vi "Tracking_SavePoint.vi"(8 "error in":errorcluster, 10 "Image Data":T4 {"Frame Data"."Image Type" items=["Grayscale (U8)", "Grayscale (I16)", "Grayscale (SGL)", "Complex (CSG)", "RGB (U32)", "HSL (U32)", "RGB (U64)", "Grayscale (U16)"]}, 11 "Recording Data In":T1) -> (0 "error out":errorcluster)   [LabVIEW 2017, in "ImageAcquisitionLibrary.lvlib"]
uses:
  ImageAcquisitionLibrary.lvlib
  Acquisition/AcquireData.ctl
  Recording/RecordingData.ctl
  <vilib>/vision/Image Controls.llb/IMAQ Image.ctl
  <vilib>/vision/Avi.llb/IMAQ AVI2 Refnum.ctl
  <vilib>/Utility/file.llb/Write To Spreadsheet File (DBL).vi
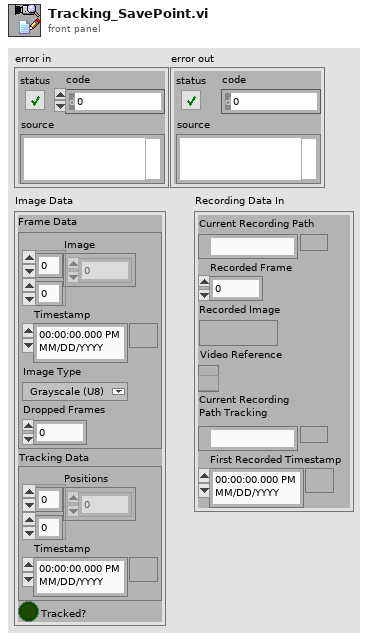
[diagram p1: front panel]
types:
  T1 = typedef "ImageAcquisitionLibrary.lvlib/RecordingData.ctl" = cluster{"Current Recording Path":path, "Recorded Frame":i32, "Recorded Image":T2, "Video Reference":T3, "Current Recording \nPath Tracking":path, "First Recorded Timestamp":timestamp}
  T2 = typedef "IMAQ Image.ctl" = refnum<image>
  T3 = typedef "IMAQ AVI2 Refnum.ctl" = refnum<k20>
  T4 = typedef "ImageAcquisitionLibrary.lvlib/AcquireData.ctl" = cluster{"Frame Data":cluster{"Image":u32[][], "Timestamp":timestamp, "Image Type":T5, "Dropped Frames":u32}, "Tracking Data":cluster{"Positions":dbl[][], "Timestamp":timestamp}, "Tracked?":bool}
  T5 = typedef "Image Type" = u32
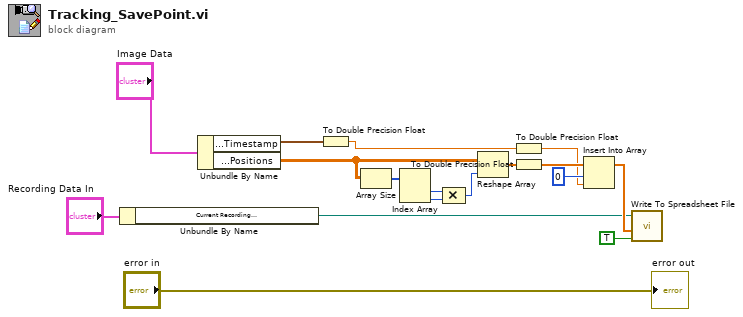
[diagram p0: block diagram]
diagram:
  n1 = Unbundle By Name("Recording Data In") -> ("Current Recording \nPath Tracking"=w3:path)
  n2 = Unbundle By Name("Image Data") -> ("Frame Data.Timestamp"=w2:timestamp, "Tracking Data.Positions"=w12:dbl[][])
  n3 = To Double Precision Float(number=w2) -> (double precision float=w1:dbl)
  n4 = Array Size(array=w12) -> (size(s)=w17:i32[])
  n5 = Index Array(array=w17) -> (element #1=w16:i32, element #2=w15:i32)  [unwired: 2 in]
  n6 = Compound Arithmetic op=MULTIPLY(w16, w15) -> (w14:i32)
  n7 = Reshape Array(w12, w14) -> (w10:dbl[])
  n8 = To Double Precision Float(number=w1) -> (double precision float=w8:dbl)
  n9 = To Double Precision Float(number=w10) -> (double precision float=w9:dbl[])
  n10 = Insert Into Array(array=w9, index=0, new element=w8) -> (w7:dbl[])
  n11 = call-poly <vilib>:"Write To Spreadsheet File.vi"("append to file? (new file:F)"=TRUE, "1D data"=w7, "file path (dialog if empty)"=w3) -> ()  [unwired: 5 in, 1 out]
  "error out" <- "error in"
